vi "VII Slave Read Bytes.vi"(9 "I2CIndex":i32, 10 "DevIndex":i32, 11 "DevType":i32) -> (1 "function return":i32, 2 "pLen":u16, 3 "pReadData":u8[](array[numeric]))   [LabVIEW 2010, in "ControlI2C.lvlib"]
doc: "int __stdcall VII_SlaveReadBytes(int DevType,int DevIndex,int I2CIndex,unsigned char* pReadData,unsigned short *pLen);"
uses:
  ControlI2C.lvlib
  ControlI2C/Ginkgo_Driver.dll
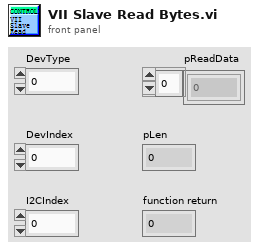
[diagram p1: front panel]
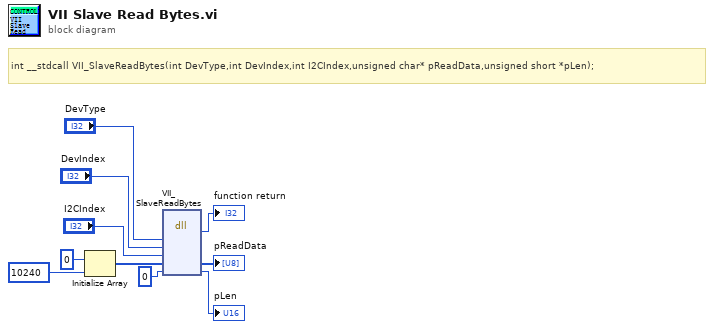
[diagram p0: block diagram]
diagram:
  # "int __stdcall VII_SlaveReadBytes(int DevType,int DevIndex,int I2CIndex,unsigned char* pReadData,unsigned short *pLen);"
  n1 = Initialize Array(u8 0 ("element"), 10240 ("dimension size")) -> (w6:u8[])
  n2 = dll-call lib="E:/Project/vt_ginkgo/truck/Ginkgo Driver/vs2010/Ginkgo_USB-I2C&SPI&CAN_API_v2.0.3.3/lib/labview_32bit/ControlI2C/Ginkgo_Driver.*" fn="VII_SlaveReadBytes"("DevType"="DevType", "DevIndex"="DevIndex", "I2CIndex"="I2CIndex", "pReadData"=w6, "pLen"=u16 0) -> (→"function return":i32, "pReadData"=→"pReadData":u8[], "pLen"=→"pLen":u16)  [unwired: 6 in, 2 out]
